vi "host_for_Tx_and_Rx_with scope.vi"() -> ()   [LabVIEW 2021]
uses:
  <vilib>/userdefined/High Color/nirio_resource_hc.ctl
  CTL/user config.ctl
  classes/5785_2_x_1600MHz/5785_2_x_1600MHz.lvclass
  <vilib>/Analysis/NI_AALBase.lvlib
  use with scope/states_for scope.ctl
  classes/device_type/device_type.lvclass
  <instrlib>/niScope/Acquire/Fetch/niScope Multi Fetch WDT.vi
  <instrlib>/niScope/Configure/Trigger/niScope Configure Trigger Edge.vi
  <vilib>/Analysis/1siggen.llb/Ramp Pattern by Delta.vi
  <instrlib>/niScope/Controls/niScope vertical coupling.ctl
  C:/Users/PXIe8108_Demo/Documents/CHAIM DATA/chaim/5785_sync_for_elbit/tx_pulse/pulse Tx Folder_lv_21/EMEA_ADG_EW_Multi_Emitter_Scenarios/classes/device_type/device_type.lvclass
  C:/Users/PXIe8108_Demo/Documents/CHAIM DATA/chaim/5785_sync_for_elbit/tx_pulse/pulse Tx Folder_lv_21/EMEA_ADG_EW_Multi_Emitter_Scenarios/classes/5785_2_x_1600MHz/5785_2_x_1600MHz.lvclass
panel:
  in  "scope cal file":path=path "C:/Users/PXIe8108_Demo/Documents/CHAIM DATA/chaim/5785_sync_for_elbit/tx_pulse/pulse Tx Folder_lv_21/EMEA_ADG_EW_Multi_Emitter_Scenarios/data/scope_cal_file.tdms"
  out "run number":i32
  in  "number of runs for test":dbl=5.0 format="%#_13g"
  in  "number of runs for cal":dbl=10.0 format="%#_13g"
  in  "read file":bool
  in  "save file":bool
  in  "file path":path=path "C:/Users/PXIe8108_Demo/Documents/CHAIM DATA/chaim/5785_sync_for_elbit/tx_pulse/pulse Tx Folder_lv_21/EMEA_ADG_EW_Multi_Emitter_Scenarios/data/cal_file.tdms"
  out "state":T1
  in  "cal":bool
  out "phase cal test (deg)":cluster{dbl[], dbl[]}[](graph)
  out "amp cal test(dB) 2":cluster{dbl[], dbl[]}[](graph)
  in  "cal mode":bool=TRUE
  in  "connection table (cannels 1,2,3 only)":dbl[](array[numeric])=[5.0, 2.0, 3.0]
  out "delta phase(deg)":cluster{dbl[], dbl[]}[](graph)
  out "delta amp (dB)":cluster{dbl[], dbl[]}[](graph)
  out "working":bool
  in  "Channel Name":string="0,1,2,3"
  in  "Resource Name":refnum<k15>="scope1" caption="Resource Name(s)"
  in  "pulse amplitude (dB)":dbl=-40.0 format="%#_13g"
  in  "pulse duration (s)":dbl=0.0002 format="%#_13p"
  in  "frequncy comb":cluster{"start":dbl, "end":dbl, "delta":dbl}={"start"=5000000.0, "end"=300000000.0, "delta"=500000.0} {"delta" format="%#_6p"; "end" format="%#_6p"; "start" format="%#_6p"}
  in  "devicess":T2[](array[typedef])=["5785_00", "5785_01", "5785_02"]
  # "5785 system alignment"
  # "RF setup"
  # "Cal Data"
  # "HW setup"
  # "scope mapping:\nchannel 0 => 5785_02 _0 \nchannel 1 => 5785_01 _0 \nchannel 2 => 5785_01 _1 \nchannel 3 => 5785_00 _1"
  # "Cal test"
  # "SW setup"
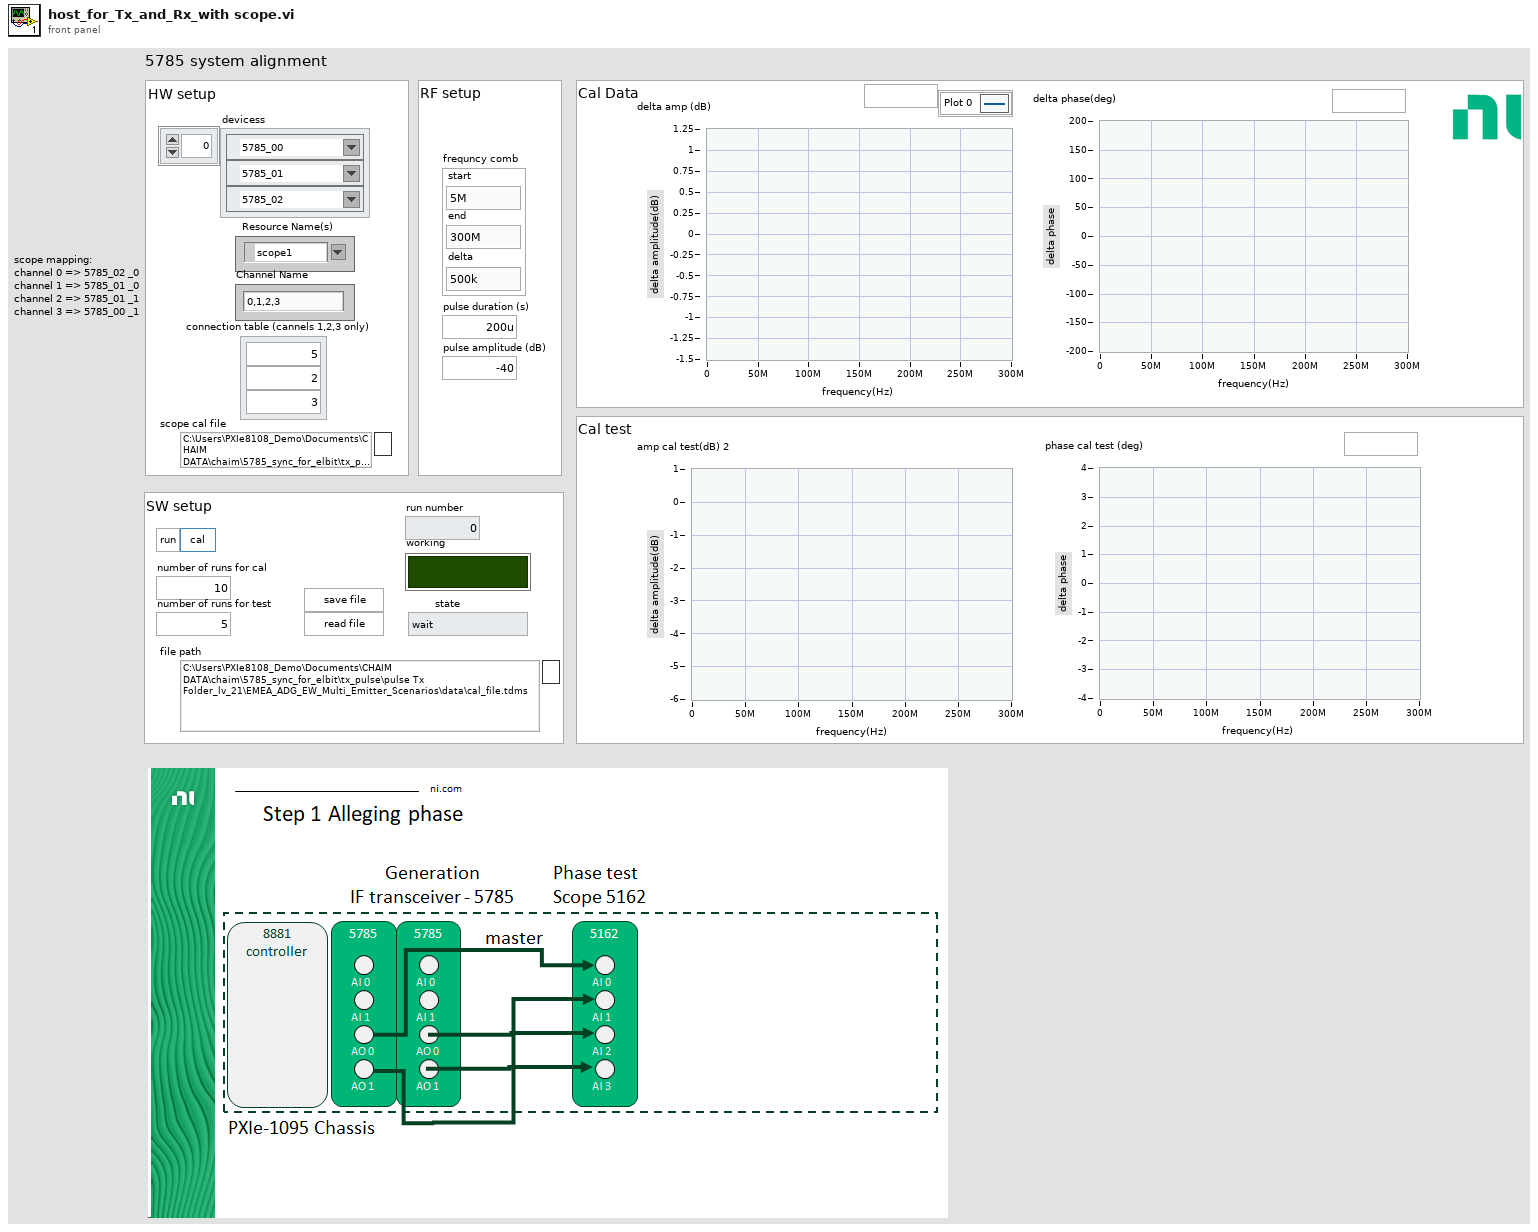
[diagram p1: front panel]
types:
  T1 = typedef "states_for scope.ctl" = enum16{"wait", "update ME config", "gen secenario", "INI ME", "INI scope", "trig", "close ME", "run mesearment", "save cal data", "get file data", "gen PDW file", "keep the data", "reset memory data", "prime the fifo"}
  T2 = typedef "nirio_resource_hc.ctl" = tag
  T3 = cluster{"freqency":dbl[], "phase":dbl[], "amp":dbl[]}
  T4 = enum16{"open", "open or create", "create or replace", "create", "open (read-only)"}
  T5 = typedef "user config.ctl" = cluster{"vst_device":refnum<k15>[], "RF gain ":dbl, "buffer size":u32, "center frequency (Hz) ":dbl, "P2P sample rate":dbl, "mode":enum16{"USRP - 180MHz", "5785 - 2*180MHz", "5785 - 3.2GHz", "P2P - VST"}, "devicess":T2[], "gen for df":bool, "Rx settings":cluster{"min PW         ":dbl, "max gap        ":dbl, "detection bar":dbl, "peak detect                        ":bool}, "use arb files":bool}
  T6 = typedef "states_for scope.ctl" = enum16{"wait", "update ME config", "gen secenario", "INI ME", "INI scope", "sync and trig", "close ME", "run mesearment", "save cal data", "get file data", "gen PDW file", "keep the data", "reset memory data"}
  T7 = cluster{"freqency":dbl[], "phase":dbl[], "amp":dbl[]}[]
  T8 = typedef "niScope vertical coupling.ctl" = i32
  T9 = typedef "PDW_lv2.ctl" = cluster{"t start":dbl, "frequency (Hz)":dbl, "duration (sec)":dbl, "mod type":T10, "mod depth":dbl, "phase (rad)":dbl[], "amp (lin)":dbl[], "trig":bool}
  T10 = typedef "mode_type.ctl" = enum8{"CW", "from memory 1", "NC - cw", "LFM", "BPSK", "QPSK"}
  T11 = typedef "PDW_lv2.ctl" = cluster{"t start":dbl, "frequency (Hz)":dbl, "duration (sec)":dbl, "mod type":T10, "mod depth":dbl, "trig":bool, "amp (lin)":dbl, "diraction (deg)":dbl, "phase(deg)":dbl}
  T12 = cluster{"frequncy":dbl, "d amp":dbl, "d phase":dbl}[]
  T13 = cluster{"frequncy":dbl, "d amp":dbl, "d phase":dbl}[][]
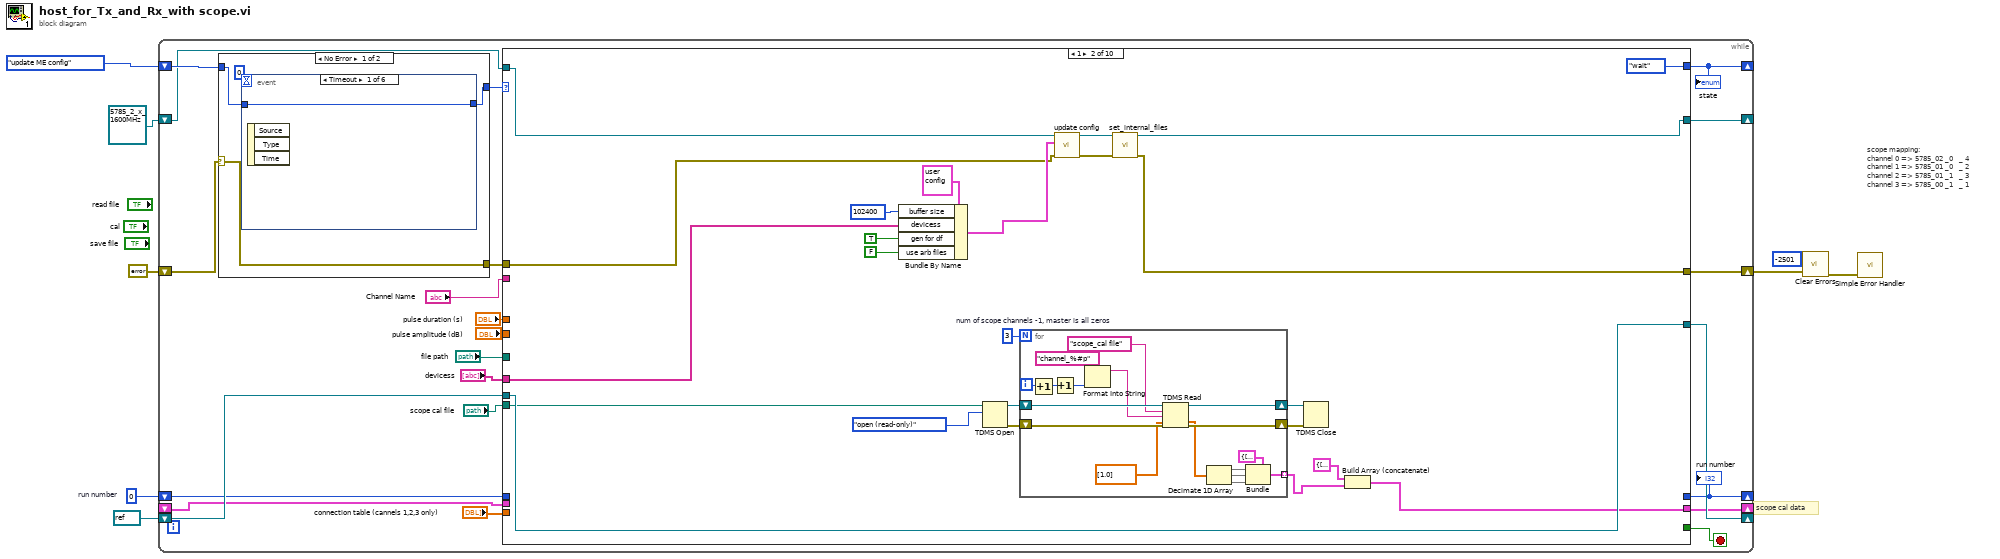
[diagram p0: block diagram]
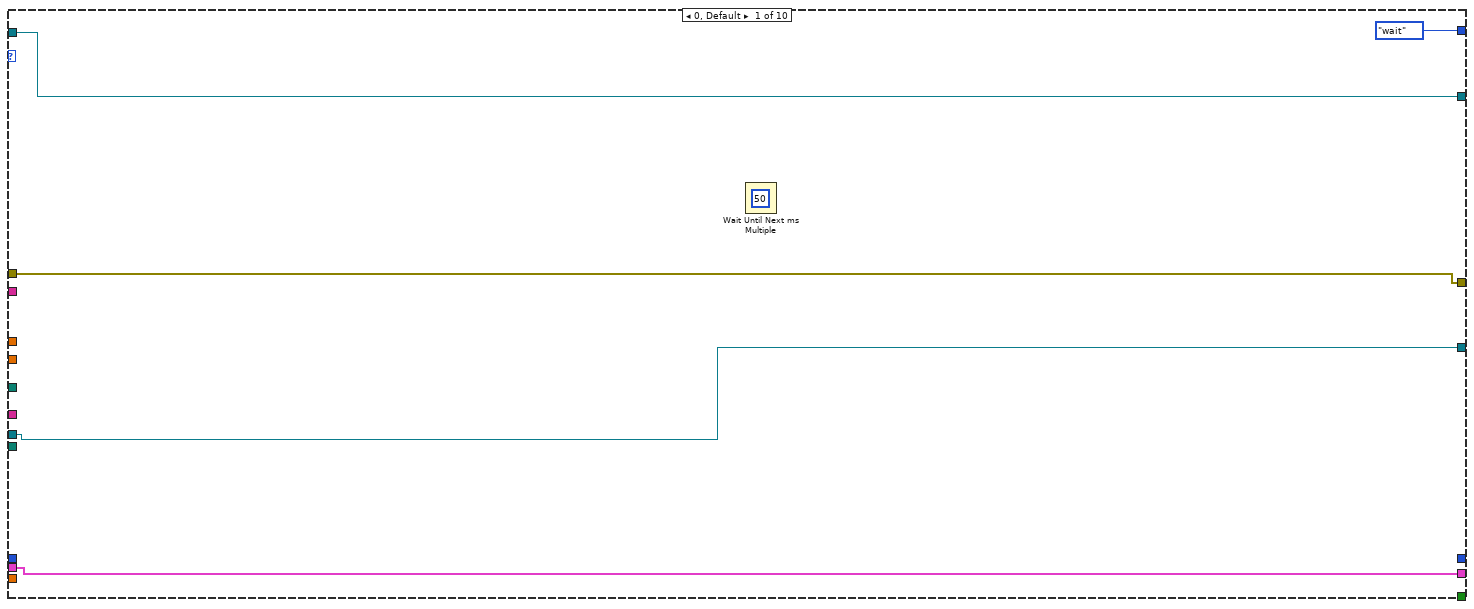
[diagram p2: hidden frame]
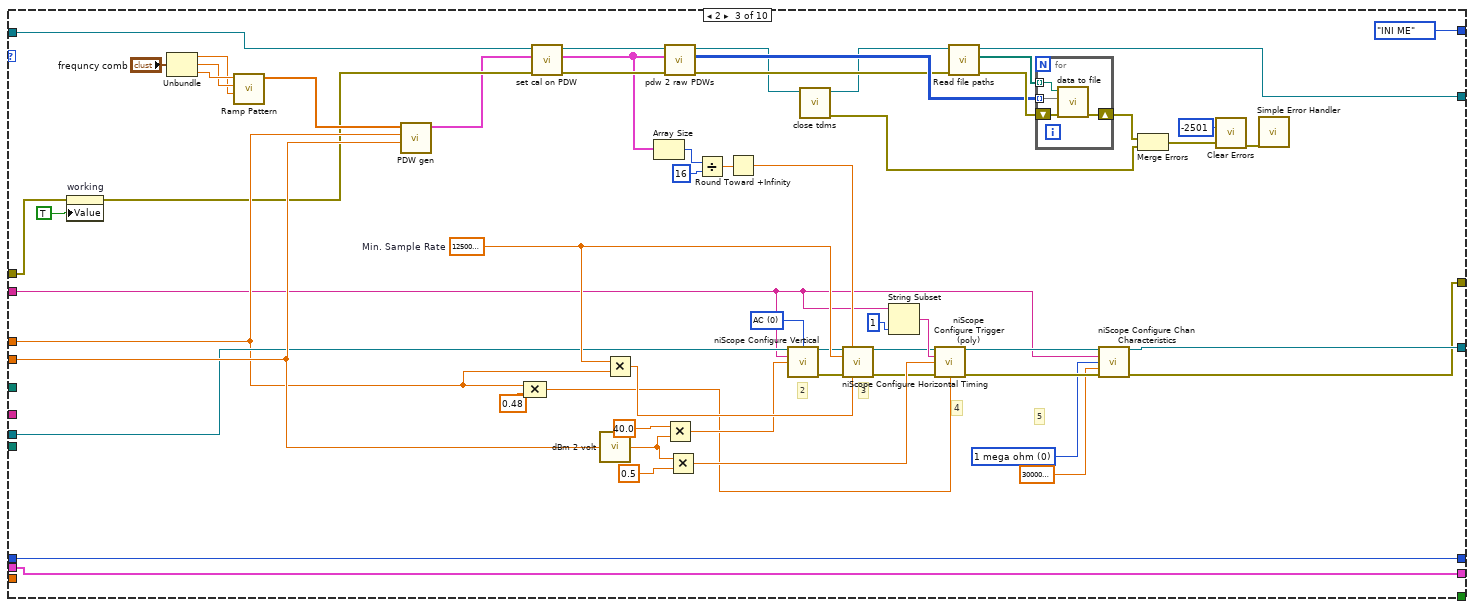
[diagram p3: hidden frame]
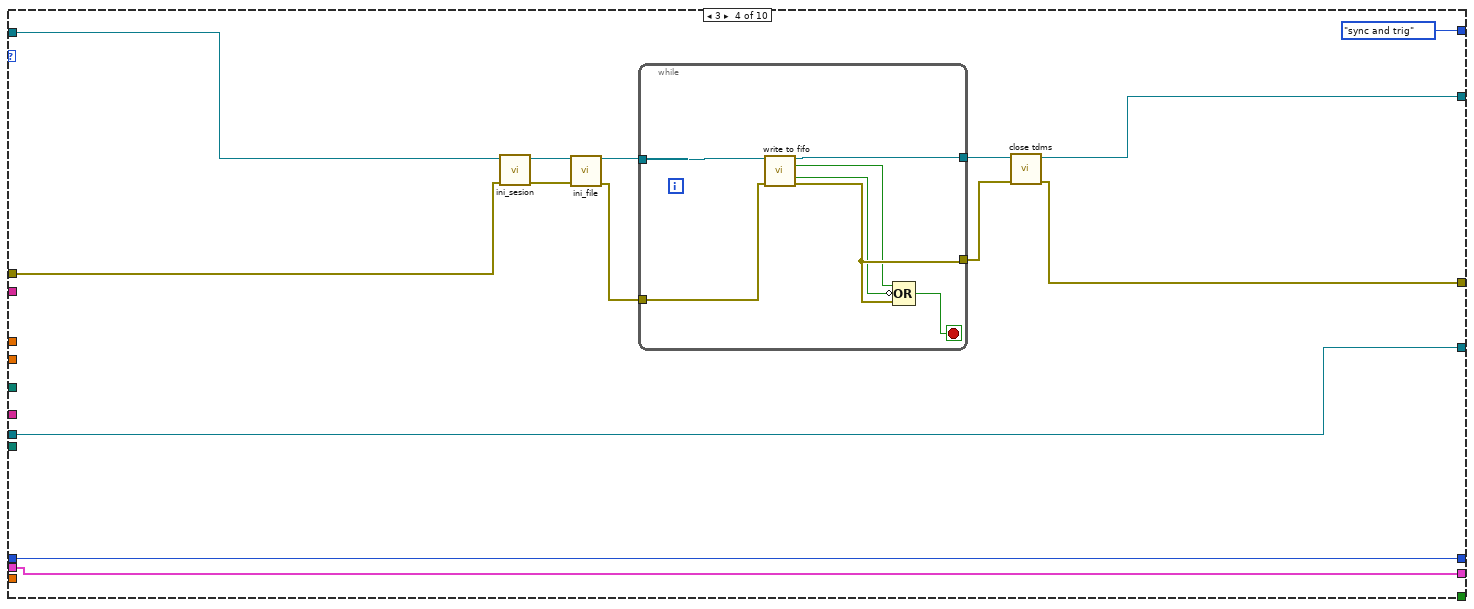
[diagram p4: hidden frame]
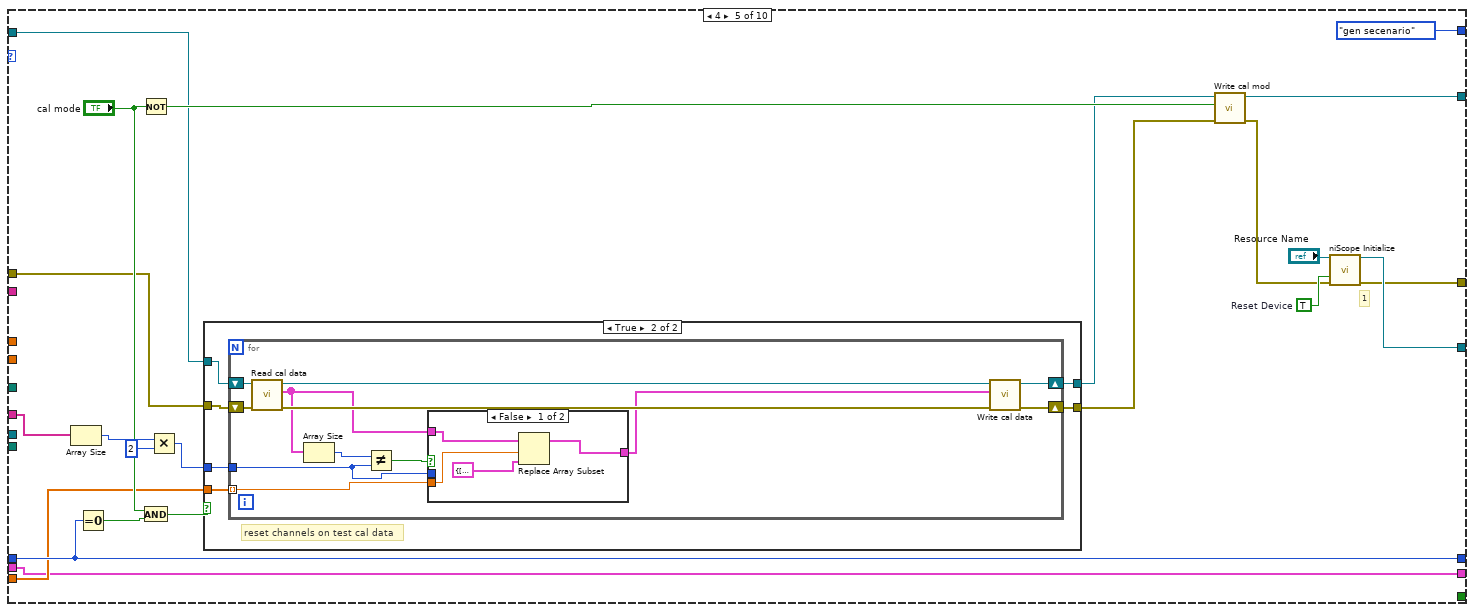
[diagram p5: hidden frame]
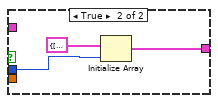
[diagram p7: hidden frame]
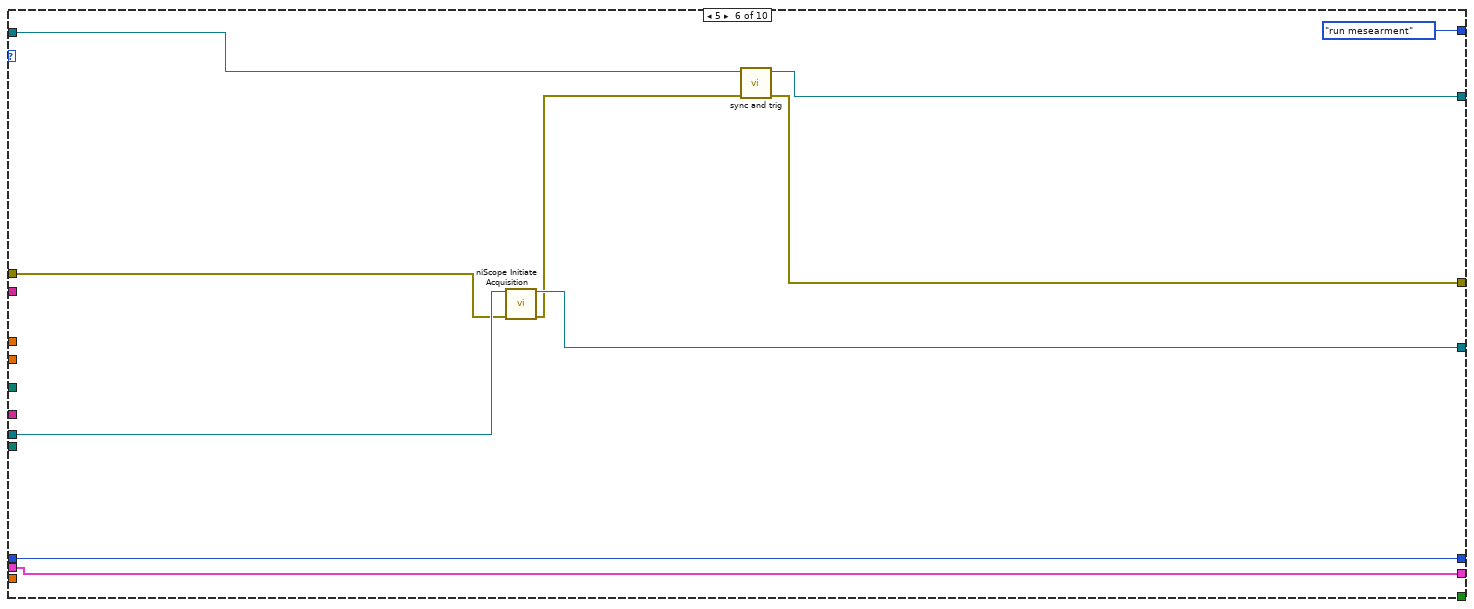
[diagram p8: hidden frame]
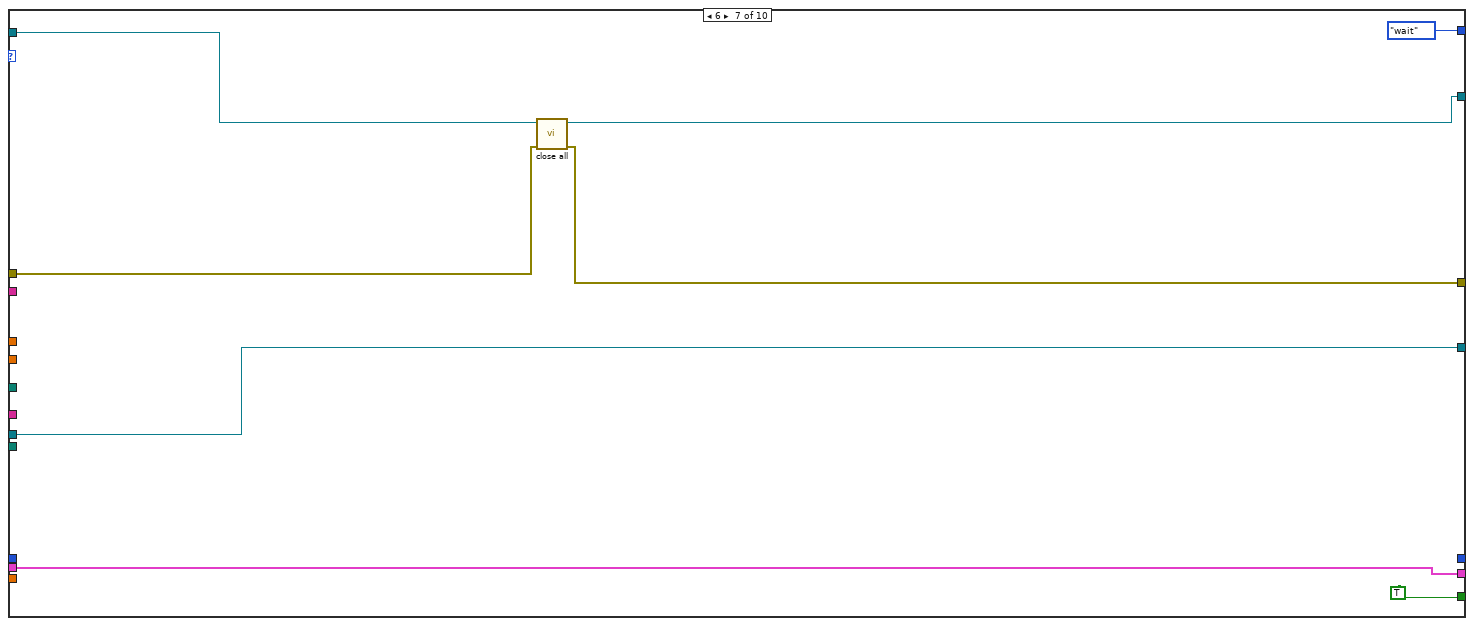
[diagram p9: hidden frame]
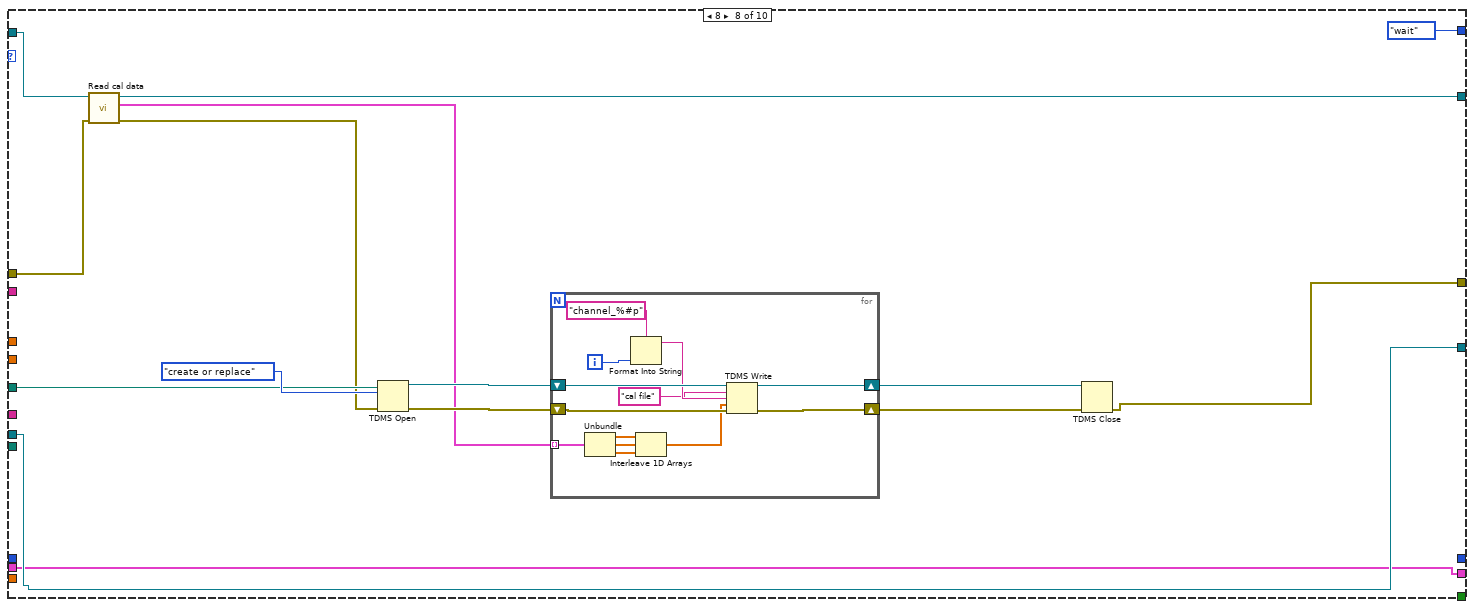
[diagram p10: hidden frame]
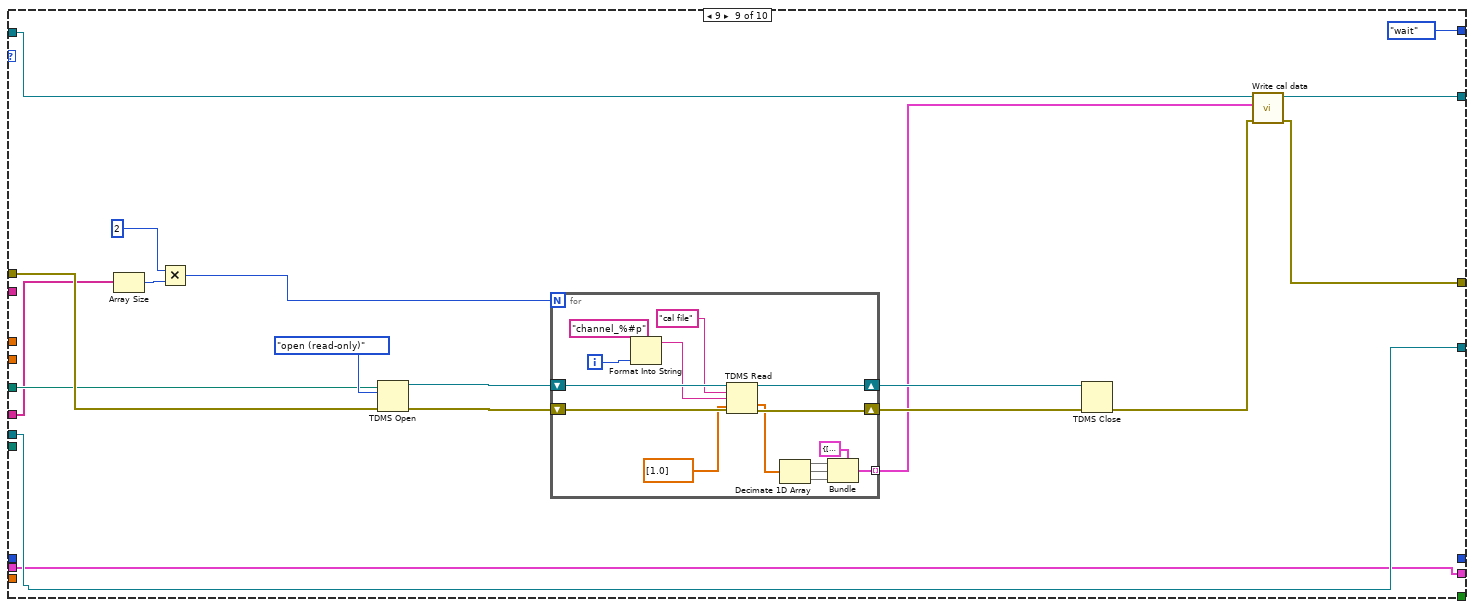
[diagram p11: hidden frame]
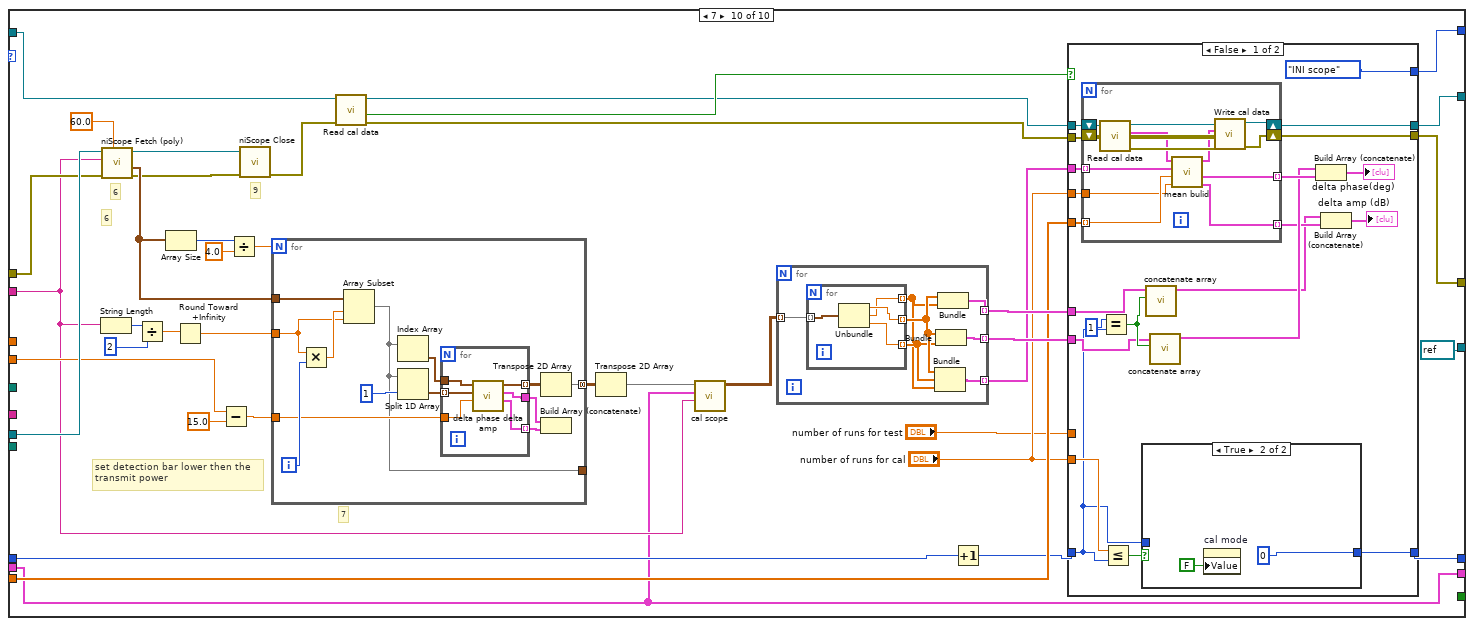
[diagram p12: hidden frame]
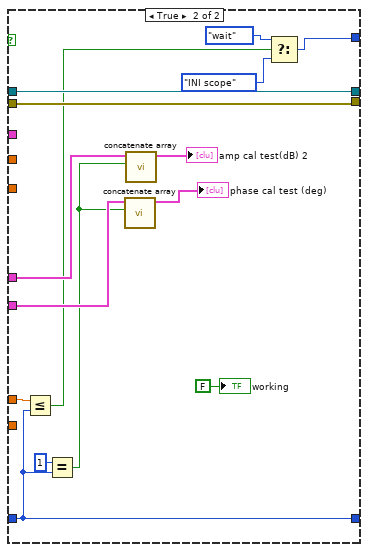
[diagram p14: hidden frame]
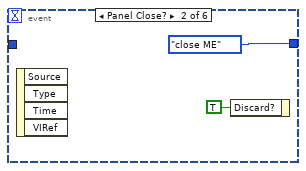
[diagram p15: hidden frame]
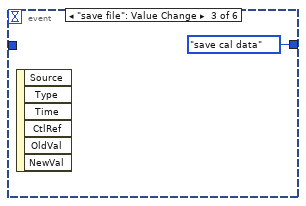
[diagram p16: hidden frame]
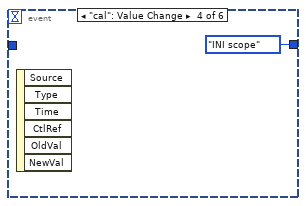
[diagram p17: hidden frame]
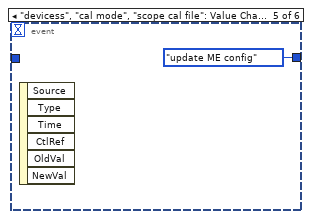
[diagram p18: hidden frame]
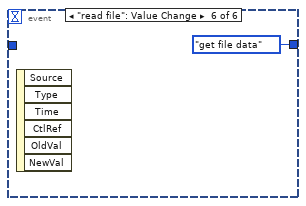
[diagram p19: hidden frame]
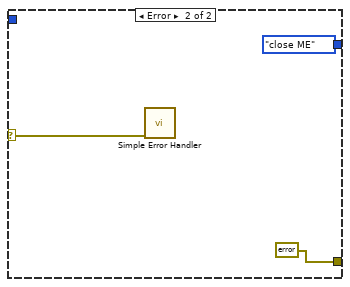
[diagram p20: hidden frame]
diagram:
  (unwired) -2501 ("specific error code to clear (0: all)")
  w3 = 0  # run number
  # "scope cal data"
  # "scope mapping:\nchannel 0 => 5785_02 _0   _ 4\nchannel 1 => 5785_01 _0   _ 2 \nchannel 2 => 5785_01 _1   _ 3\nchannel 3 => 5785_00 _1   _ 1"
  n1 = while {
    shift-right: [w16] -> _
    shift-left: states_for_scope."update ME config" -> [w27]
    shift-right: [w24] -> w2
    shift-left: errorcluster {"status"=FALSE, "code"=0, "source"=""} ("error out") -> [w29]
    shift-right: [w21] -> _
    shift-left: refnum<k15> refnum ("instrument handle out") -> [w20]
    shift-right: [w25] -> _
    shift-left: refnum<class "5785_2_x_1600MHz.lvclass"> refnum ("5785_2_x_1600MHz.lvclass") -> [w18]
    shift-right: [w12] -> _
    shift-left: w3 -> [w13]
    shift-right: [w9] -> _
    shift-left: _ -> [w8]
    stop <- w17 stop-if-true
    n2 = case shown="No Error" w29 {
      selector: w29 -> [w414 w424]
      tunnel: [w412 states_for_scope."close ME"] -> w28
      tunnel: w27 -> [w413 _]
      tunnel: [w414 errorcluster {"status"=FALSE, "code"=0, "source"=""} ("error IO")] -> w26
      frame No Error {
        n3 = event shown="[0] Timeout" {
          selector: _ -> [_ _ _ _ _ _]
          dyn-events: _ -> [_ _ _ _ _ _]
          timeout: 0 -> [_ _ _ _ _ _]
          tunnel: w413 -> [w415 _ _ _ _ _]
          tunnel: [w415 states_for_scope."close ME" states_for_scope."save cal data" states_for_scope."INI scope" states_for_scope."update ME config" states_for_scope."get file data"] -> w412
          event Timeout {
            n4 = event-data() -> ()  [unwired: 1 in, 3 out]
          }
          event Panel Close? {
            n5 = event-data() -> ()  [unwired: 1 in, 4 out]
            n6 = event-data("Discard?"=TRUE) -> ()  [unwired: 1 in, 1 out]
          }
          event "save file": Value Change {
            n7 = event-data() -> ()  [unwired: 1 in, 6 out]
          }
          event "cal": Value Change {
            n8 = event-data() -> ()  [unwired: 1 in, 6 out]
          }
          event "devicess", "cal mode", "scope cal file": Value Change {
            n9 = event-data() -> ()  [unwired: 1 in, 6 out]
          }
          event "read file": Value Change {
            n10 = event-data() -> ()  [unwired: 1 in, 6 out]
          }
        }
      }
      frame Error {
        n11 = call <vilib>:"Simple Error Handler.vi"("error in (no error)"=w424) -> ()  [unwired: 4 in, 5 out]
      }
    }
    n12 = case shown="1" w28 {
      tunnel: w26 -> [w33 w50 w98 w147 w167 w214 w224 w229 w270 w316]
      tunnel: [w34 w48 w105 w140 w175 w212 w225 w231 w259 w308] -> w25
      tunnel: [w33 w47 w86 w141 w178 w215 w223 w235 w256 w310] -> w24
      tunnel: "pulse duration (s)" -> [_ _ w106 _ _ _ _ _ _ _]
      tunnel: "pulse amplitude (dB)" -> [_ _ w108 _ _ _ _ _ _ w311]
      tunnel: [w32 w52 w87 w146 w179 w217 w222 w240 w272 refnum<k15> refnum ("instrument handle out")] -> w21
      tunnel: w20 -> [w32 w52 w107 w146 _ w218 w222 w240 w272 w317]
      tunnel: "Channel Name" -> [_ _ w83 _ _ _ _ _ _ w290]
      tunnel: w18 -> [w34 w46 w95 w148 w172 w213 w226 w232 w260 w309]
      tunnel: [_ _ _ _ _ _ TRUE _ _ _] -> w17
      tunnel: [states_for_scope."wait" states_for_scope."wait" states_for_scope."INI ME" states_for_scope."sync and trig" states_for_scope."gen secenario" states_for_scope."run mesearment" states_for_scope."wait" states_for_scope."wait" states_for_scope."wait" w303] -> w16
      tunnel: "file path" -> [_ _ _ _ _ _ _ w233 w265 _]
      tunnel: "devicess" -> [_ w49 _ _ w163 _ _ _ w262 _]
      tunnel: w13 -> [_ _ w91 w144 w173 w210 _ _ _ w298]
      tunnel: [_ _ w91 w144 w173 w210 _ _ _ w300] -> w12
      tunnel: "connection table (cannels 1,2,3 only)" -> [_ _ _ _ w165 _ _ _ _ w302]
      tunnel: "scope cal file" -> [_ w39 _ _ _ _ _ _ _ _]
      tunnel: [w30 w36 w77 w139 w164 w209 w219 w227 w255 w289] -> w9
      tunnel: w8 -> [w30 _ w77 w139 w164 w209 w219 w227 w255 w289]
      frame 0, Default {
        n13 = Wait Until Next ms Multiple(millisecond multiple=u32 50) -> ()  [unwired: 1 out]
      }
      frame 1 {
        w41 = 3  # num of scope channels -1, master is all zeros
        n14 = Bundle By Name(cluster=T5 {"vst_device"=["VST_1", "VST_2"], "RF gain "=10.0, "buffer size"=524288, "center frequency (Hz) "=1000000000.0, "P2P sample rate"=200000000.0, "mode"=enum."5785 - 2*180MHz", "devicess"=["IF_transiver_0", "IF_transiver_1", "IF_transiver_2"], "gen for df"=FALSE, "Rx settings"={"min PW         "=0.0, "max gap        "=0.0, "detection bar"=0.0, "peak detect                        "=FALSE}, "use arb files"=TRUE} ("user configurations"), "buffer size"=u32 102400, "devicess"=w49, "gen for df"=TRUE, "use arb files"=FALSE) -> (w59:T5)
        n15 = TDMS Open(10:T4."open (read-only)" ("operation (0:open)"), 11:w39) -> (0:w43:errorcluster, 3:w42:refnum<k34>)  [unwired: 5 in]
        n16 = for {
          N: w41 -> [_]
          shift-right: [w74] -> w44
          shift-left: w42 -> [w76]
          shift-right: [w73] -> w45
          shift-left: w43 -> [w75]
          tunnel: [w63] -> w38 mode=indexing
          i -> [w62]
          n17 = Increment(x=w62) -> (x+1=w60:i32)
          n18 = Increment(x=w60) -> (x+1=w61:i32)
          n19 = Format Into String(format string="channel_%#p", w61) -> (resulting string=w71:string)  [unwired: 2 in, 1 out]
          n20 = TDMS Read(0:w76, 5:"scope_cal file" ("group name in (Untitled)"), 7:w71, 11:w75, 12:dbl[] [1.0] ("interleaved array")) -> (4:w74:refnum<k34>, 10:w68:dbl[], 15:w73:errorcluster)  [unwired: 3 in, 3 out]
          n21 = Decimate 1D Array(w68) -> (w66:dbl[], w65:dbl[], w64:dbl[])
          n22 = Bundle(cluster=T3 {"freqency"=[], "phase"=[], "amp"=[]}, "freqency"=w66, "phase"=w65, "amp"=w64) -> (w63:T3)
        }
        n23 = call-dynamic "update config.vi"("error in (no error)"=w50, "user configurations"=w59, "5785_2_x_1600MHz in"=w46) -> ("error out"=w57:errorcluster, "5785_2_x_1600MHz out"=w58:refnum<class "5785_2_x_1600MHz.lvclass">)  [unwired: 5 in, 2 out]
        n24 = call-dynamic "set_internal_files.vi"("error in (no error)"=w57, "device_type in"=w58) -> ("error out"=w47:errorcluster, "device_type out"=w48:refnum<class "5785_2_x_1600MHz.lvclass">)  [unwired: 8 in]
        n25 = TDMS Close(8:w45, 11:w44) -> ()  [unwired: 2 out]
        n26 = Build Array (concatenate)(T3 {"freqency"=[], "phase"=[], "amp"=[]}, w38) -> (w36:T7)
      }
      frame 2 {
        w85 = u32 0 items=["1 mega ohm"=0, "50 ohms"=2] ("input impedance")
        w90 = T8 0 items=["AC", "DC", "Ground"] ("vertical coupling")
        w114 = 1250000000.0  # Min. Sample Rate
        # "5"
        # "4"
        # "3"
        # "2"
        n27 = property on="working" class="Bool (strict)"(error in=w98, "Value"=TRUE ("done")) -> (error out=w94:errorcluster)  [unwired: 1 in, 1 out]
        n28 = Unbundle("frequncy comb") -> ("start"=w129:dbl, "end"=w130:dbl, "delta"=w131:dbl)
        n29 = call-poly <vilib>:"Ramp Pattern.vi"("start"=w129, "end"=w130, "delta"=w131) -> ("Ramp Pattern"=w132:dbl[])  [unwired: 6 in, 2 out]
        n30 = call "PDW gen.vi"("pulse amplitude"=w108, "pulse duration"=w106, "frequency list"=w132) -> ("PDW out"=w93:T9[])  [unwired: 7 in, 1 out]
        n31 = Compound Arithmetic op=MULTIPLY(w106, 0.48 ("value")) -> (w118:dbl)
        n32 = call "set cal on PDW.vi"("error in (no error)"=w94, "PDWs on channels"=w93, "device_type in"=w95) -> ("error out"=w96:errorcluster, "PDWs on channels"=w92:cluster{T11[]}[], "device_type out"=w97:refnum<class "5785_2_x_1600MHz.lvclass">)  [unwired: 6 in]
        n33 = call "dBm 2 volt.vi"("dBm"=w108) -> ("V"=w119:dbl)
        n34 = Multiply(x=w114, y=w106) -> (x*y=w122:dbl)
        n35 = Array Size(array=w92) -> (size(s)=w133:i32)
        n36 = call-dynamic "pdw 2 raw PDWs.vi"("error in (no error)"=w96, "PDWs on channels"=w92, "device_type in"=w97) -> ("error out"=w124:errorcluster, "Array"=w126:u64[][], "device_type out"=w101:refnum<class "5785_2_x_1600MHz.lvclass">)  [unwired: 6 in]
        n37 = Multiply(x=40.0, y=w119) -> (x*y=w121:dbl)
        n38 = Multiply(x=w119, y=0.5) -> (x*y=w120:dbl)
        n39 = Divide(x=w133, y=16) -> (x/y=w134:dbl)
        n40 = Round Toward +Infinity(x=w134) -> (ceil(x): smallest int >= x=w109:dbl)
        n41 = call <instrlib>:"niScope Configure Vertical.vi"("instrument handle"=w107, "vertical coupling"=w90, "channels"=w83, "vertical range"=w121) -> ("instrument handle out"=w103:refnum<k15>, "error out"=w102:errorcluster)  [unwired: 10 in]
        n42 = call-dynamic "close tdms.vi"("device_type in"=w101) -> ("error out"=w80:errorcluster, "device_type out"=w100:refnum<class "5785_2_x_1600MHz.lvclass">)  [unwired: 9 in]
        n43 = call <instrlib>:"niScope Configure Horizontal Timing.vi"("instrument handle"=w103, "number of records"=w109, "min sample rate"=w114, "error in"=w102, "min record length"=w122) -> ("instrument handle out"=w116:refnum<k15>, "error out"=w115:errorcluster)  [unwired: 9 in]
        n44 = String Subset(string=w83, length (rest)=1 ("length (rest)")) -> (substring=w117:string)  [unwired: 1 in]
        n45 = call-poly <instrlib>:"niScope Configure Trigger (poly).vi"("instrument handle"=w116, "trigger source"=w117, "trigger level"=w120, "error in"=w115, "trigger delay"=w118) -> ("instrument handle out"=w89:refnum<k15>, "error out"=w88:errorcluster)  [unwired: 9 in]
        n46 = call-dynamic "Read file paths.vi"("error in (no error)"=w124, "device_type in"=w100) -> ("error out"=w127:errorcluster, "file paths"=w125:path[], "device_type out"=w105:refnum<class "5785_2_x_1600MHz.lvclass">)  [unwired: 6 in, 1 out]
        n47 = for {
          tunnel: w126 -> [w136] mode=indexing
          shift-right: [w137] -> w81
          shift-left: w127 -> [w138]
          tunnel: w125 -> [w135] mode=indexing
          n48 = call "data to file.vi"("error in (no error)"=w138, "Array"=w136, "Path"=w135) -> ("error out"=w137:errorcluster)  [unwired: 8 in]
        }
        n49 = call <instrlib>:"niScope Configure Chan Characteristics.vi"("instrument handle"=w89, "channels"=w83, "input impedance"=w85, "maximum input frequency"=300000000.0, "error in"=w88) -> ("instrument handle out"=w87:refnum<k15>, "error out"=w86:errorcluster)  [unwired: 9 in]
        n50 = Merge Errors(w81, w80) -> (w79:errorcluster)
        n51 = call <vilib>:"Clear Errors.vi"("error in (no error)"=w79, "specific error code to clear (0: all)"=-2501) -> ("error out"=w78:errorcluster)  [unwired: 4 in, 1 out]
        n52 = call <vilib>:"Simple Error Handler.vi"("error in (no error)"=w78) -> ()  [unwired: 4 in, 5 out]
      }
      frame 3 {
        n53 = call-dynamic "ini_sesion.vi"("error in (no error)"=w147, "5785_2_x_1600MHz in"=w148) -> ("error out"=w150:errorcluster, "5785_2_x_1600MHz out"=w149:refnum<class "5785_2_x_1600MHz.lvclass">)  [unwired: 8 in]
        n54 = call-dynamic "ini_file.vi"("device_type in"=w149, "error in (no error)"=w150) -> ("device_type out"=w151:refnum<class "5785_2_x_1600MHz.lvclass">, "error out"=w152:errorcluster)  [unwired: 11 in, 1 out]
        n55 = while {
          tunnel: w151 -> [w159]
          tunnel: w152 -> [w158]
          tunnel: [w157] -> w143
          tunnel: [w155] -> w142
          stop <- w156 stop-if-true
          n56 = call-dynamic "write to fifo.vi"("5785_2_x_1600MHz in"=w159, "error in (no error)"=w158) -> ("5785_2_x_1600MHz out"=w157:refnum<class "5785_2_x_1600MHz.lvclass">, "done write file"=w153:bool, "room on fifo"=w154:bool, "error out"=w155:errorcluster)  [unwired: 9 in, 1 out]
          n57 = Compound Arithmetic op=OR(w153, invert w154, w155) -> (w156:bool)
        }
        n58 = call-dynamic "close tdms.vi"("error in (no error)"=w142, "device_type in"=w143) -> ("error out"=w141:errorcluster, "device_type out"=w140:refnum<class "5785_2_x_1600MHz.lvclass">)  [unwired: 8 in]
      }
      frame 4 {
        w180 = TRUE  # Reset Device
        # "1"
        n59 = Array Size(array=w163) -> (size(s)=w162:i32)
        n60 = Equal To 0?(x=w173) -> (x = 0?=w169:bool)
        n61 = Not(x="cal mode") -> (.not. x?=w176:bool)
        n62 = And(x="cal mode", y=w169) -> (x .and. y?=w168:bool)
        n63 = Multiply(x=w162, y=2) -> (x*y=w160:i32)
        n64 = case shown="True" w168 {
          tunnel: w172 -> [w183 w189]
          tunnel: [w183 w188] -> w171
          tunnel: w167 -> [w182 w187]
          tunnel: [w182 w186] -> w166
          tunnel: w165 -> [_ w185]
          tunnel: w160 -> [_ w184]
          frame False {
          }
          frame True {
            # "reset channels on test cal data"
            n65 = for {
              shift-right: [w198] -> w188
              shift-left: w189 -> [w199]
              shift-right: [w196] -> w186
              shift-left: w187 -> [w197]
              tunnel: w185 -> [w191] mode=indexing
              tunnel: w184 -> [w190]
              n66 = call-dynamic "Read cal data.vi"("error in (no error)"=w197, "device_type in"=w199) -> ("error out"=w200:errorcluster, "cal data"=w194:T7, "device_type out"=w201:refnum<class "5785_2_x_1600MHz.lvclass">)  [unwired: 6 in, 1 out]
              n67 = Array Size(array=w194) -> (size(s)=w193:i32)
              n68 = Not Equal?(x=w193, y=w190) -> (x != y?=w192:bool)
              n69 = case shown="False" w192 {
                tunnel: w194 -> [w205 _]
                tunnel: [w204 w208] -> w195
                tunnel: w191 -> [w203 _]
                tunnel: w190 -> [_ w206]
                frame False {
                  n70 = Replace Array Subset(array=w205, new element=T3 {"freqency"=[], "phase"=[], "amp"=[]} ("new element/subarray"), index=w203) -> (w204:T7)
                }
                frame True {
                  n71 = Initialize Array(cluster{dbl[], dbl[], dbl[]} {[], [], []} ("new element/subarray"), w206) -> (w208:cluster{dbl[], dbl[], dbl[]}[])
                }
              }
              n72 = call-dynamic "Write cal data.vi"("error in (no error)"=w200, "cal data"=w195, "device_type in"=w201) -> ("error out"=w196:errorcluster, "device_type out"=w198:refnum<class "5785_2_x_1600MHz.lvclass">)  [unwired: 7 in]
            }
          }
        }
        n73 = call-dynamic "Write cal mod.vi"("error in (no error)"=w166, "apply cal data"=w176, "device_type in"=w171) -> ("error out"=w174:errorcluster, "device_type out"=w175:refnum<class "5785_2_x_1600MHz.lvclass">)  [unwired: 7 in]
        n74 = call <instrlib>:"niScope Initialize.vi"("resource name"="Resource Name", "reset device"=w180, "error in"=w174) -> ("instrument handle"=w179:refnum<k15>, "error out"=w178:errorcluster)  [unwired: 11 in]
      }
      frame 5 {
        n75 = call <instrlib>:"niScope Initiate Acquisition.vi"("instrument handle"=w218, "error in"=w214) -> ("instrument handle out"=w217:refnum<k15>, "error out"=w216:errorcluster)  [unwired: 12 in]
        n76 = call-dynamic "sync and trig.vi"("error in (no error)"=w216, "device_type in"=w213) -> ("error out"=w215:errorcluster, "device_type out"=w212:refnum<class "5785_2_x_1600MHz.lvclass">)  [unwired: 8 in]
      }
      frame 6 {
        n77 = call-dynamic "close all.vi"("error in (no error)"=w224, "5785_2_x_1600MHz in"=w226) -> ("error out"=w223:errorcluster, "5785_2_x_1600MHz out"=w225:refnum<class "5785_2_x_1600MHz.lvclass">)  [unwired: 8 in]
      }
      frame 8 {
        n78 = call-dynamic "Read cal data.vi"("error in (no error)"=w229, "device_type in"=w232) -> ("error out"=w228:errorcluster, "cal data"=w230:T7, "device_type out"=w231:refnum<class "5785_2_x_1600MHz.lvclass">)  [unwired: 6 in, 1 out]
        n79 = TDMS Open(8:w228, 10:T4."create or replace" ("operation (0:open)"), 11:w233) -> (0:w238:errorcluster, 3:w239:refnum<k34>)  [unwired: 4 in]
        n80 = for {
          shift-right: [w252] -> w237
          shift-left: w239 -> [w254]
          shift-right: [w251] -> w236
          shift-left: w238 -> [w253]
          tunnel: w230 -> [w245] mode=indexing
          i -> [w249]
          n81 = Unbundle(w245) -> ("freqency"=w244:dbl[], "phase"=w243:dbl[], "amp"=w242:dbl[])
          n82 = Format Into String(format string="channel_%#p", w249) -> (resulting string=w247:string)  [unwired: 2 in, 1 out]
          n83 = Interleave 1D Arrays(w244, w243, w242) -> (w250:dbl[])
          n84 = TDMS Write(0:w254, 5:"cal file" ("group name in (Untitled)"), 7:w247, 9:w250, 11:w253) -> (4:w252:refnum<k34>, 15:w251:errorcluster)  [unwired: 1 in, 2 out]
        }
        n85 = TDMS Close(8:w236, 11:w237) -> (0:w235:errorcluster)  [unwired: 1 out]
      }
      frame 9 {
        n86 = Array Size(array=w262) -> (size(s)=w264:i32)
        n87 = Multiply(x=2, y=w264) -> (x*y=w261:i32)
        n88 = TDMS Open(8:w270, 10:T4."open (read-only)" ("operation (0:open)"), 11:w265) -> (0:w269:errorcluster, 3:w271:refnum<k34>)  [unwired: 4 in]
        n89 = for {
          N: w261 -> [_]
          shift-right: [w286] -> w268
          shift-left: w271 -> [w288]
          shift-right: [w285] -> w267
          shift-left: w269 -> [w287]
          tunnel: [w274] -> w258 mode=indexing
          i -> [w284]
          n90 = Format Into String(format string="channel_%#p", w284) -> (resulting string=w282:string)  [unwired: 2 in, 1 out]
          n91 = TDMS Read(0:w288, 5:"cal file" ("group name in (Untitled)"), 7:w282, 11:w287, 12:dbl[] [1.0] ("interleaved array")) -> (4:w286:refnum<k34>, 10:w279:dbl[], 15:w285:errorcluster)  [unwired: 3 in, 3 out]
          n92 = Decimate 1D Array(w279) -> (w277:dbl[], w276:dbl[], w275:dbl[])
          n93 = Bundle(cluster=T3 {"freqency"=[], "phase"=[], "amp"=[]}, "freqency"=w277, "phase"=w276, "amp"=w275) -> (w274:T3)
        }
        n94 = TDMS Close(8:w267, 11:w268) -> (0:w257:errorcluster)  [unwired: 1 out]
        n95 = call-dynamic "Write cal data.vi"("error in (no error)"=w257, "cal data"=w258, "device_type in"=w260) -> ("error out"=w256:errorcluster, "device_type out"=w259:refnum<class "5785_2_x_1600MHz.lvclass">)  [unwired: 7 in]
      }
      frame 7 {
        # "set detection bar lower then the\ntransmit power"
        # "6"
        # "9"
        # "7"
        # "6"
        n96 = String Length(string=w290) -> (length=w296:i32)
        n97 = call-poly <instrlib>:"niScope Fetch (poly).vi"("timeout"=60.0, "error in"=w316, "channels"=w290, "instrument handle"=w317) -> ("error out"=w322:errorcluster, "wfm"=w326:waveform(dbl)[], "instrument handle out"=w321:refnum<k15>)  [unwired: 4 in, 1 out]
        n98 = Divide(x=w296, y=2) -> (x/y=w294:dbl)
        n99 = Array Size(array=w326) -> (size(s)=w323:i32)
        n100 = Round Toward +Infinity(x=w294) -> (ceil(x): smallest int >= x=w293:dbl)
        n101 = Subtract(x=w311, y=15.0) -> (x-y=w325:dbl)
        n102 = Divide(x=w323, y=4.0) -> (x/y=w324:dbl)
        n103 = call <instrlib>:"niScope Close.vi"("instrument handle"=w321, "error in"=w322) -> ("error out"=w307:errorcluster)  [unwired: 13 in]
        n104 = for {
          N: w324 -> [_]
          tunnel: w326 -> [w393]
          tunnel: w325 -> [w387]
          tunnel: [w385] -> w327 mode=concatenating
          tunnel: [w384] -> _
          tunnel: w293 -> [w381]
          i -> [w392]
          n105 = Multiply(x=w381, y=w392) -> (x*y=w391:dbl)
          n106 = Array Subset(array=w393, index=w391, length=w381) -> (w384:waveform(dbl)[])
          n107 = Index Array(array=w384) -> (element=w389:waveform(dbl))  [unwired: 1 in]
          n108 = Split 1D Array(array=w384, index=1) -> (second subarray=w388:waveform(dbl)[])  [unwired: 1 out]
          n109 = for {
            tunnel: w389 -> [w399]
            tunnel: w388 -> [w398] mode=indexing
            tunnel: w387 -> [w397]
            tunnel: [w396] -> w386 mode=indexing
            tunnel: [w395] -> w383
            tunnel: [w394] -> w382 mode=indexing
            n110 = call "delta phase delta amp.vi"("detection bar"=w397, "signal in 2"=w398, "signal in 1"=w399) -> ("PSD 1"=w394:cluster{"f0":dbl, "df":dbl, "magnitude":dbl[]}, "PSD 0"=w395:cluster{"f0":dbl, "df":dbl, "magnitude":dbl[]}, "cal data"=w396:T12)  [unwired: 6 in]
          }
          n111 = Transpose 2D Array(2D array=w386) -> (transposed array=w385:T13)
          n112 = Build Array (concatenate)(w383, w382) -> ()  [unwired: 1 out]
        }
        n113 = call-dynamic "Read cal data.vi"("error in (no error)"=w307, "device_type in"=w309) -> ("error out"=w304:errorcluster, "apply cal data"=w306:bool, "device_type out"=w305:refnum<class "5785_2_x_1600MHz.lvclass">)  [unwired: 6 in, 1 out]
        n114 = Transpose 2D Array(2D array=w327) -> (transposed array=w292:T13)
        n115 = call "cal scope.vi"("Channel Name"=w290, "scope cal data"=w289, "measured data"=w292) -> ("measured and cal data"=w291:T13)  [unwired: 8 in]
        n116 = for {
          tunnel: w291 -> [w406] mode=indexing
          tunnel: [w405] -> w314 mode=indexing
          tunnel: [w404] -> w313 mode=indexing
          tunnel: [w400] -> w312 mode=indexing
          n117 = for {
            tunnel: w406 -> [w410] mode=indexing
            tunnel: [w409] -> w403 mode=indexing
            tunnel: [w408] -> w402 mode=indexing
            tunnel: [w407] -> w401 mode=indexing
            n118 = Unbundle(w410) -> ("frequncy"=w409:dbl, "d amp"=w407:dbl, "d phase"=w408:dbl)
          }
          n119 = Bundle(w403, w402, w401) -> (w400:cluster{dbl[], dbl[], dbl[]})  [unwired: 1 in]
          n120 = Bundle(w403, w402) -> (w404:cluster{dbl[], dbl[]})  [unwired: 1 in]
          n121 = Bundle(w403, w401) -> (w405:cluster{dbl[], dbl[]})  [unwired: 1 in]
        }
        n122 = Increment(x=w298) -> (x+1=w297:i32)
        n123 = case shown="False" w306 {
          tunnel: w312 -> [w349 _]
          tunnel: w302 -> [w348 _]
          tunnel: w314 -> [w339 w377]
          tunnel: w313 -> [w337 w375]
          tunnel: w305 -> [w347 w379]
          tunnel: w304 -> [w346 w378]
          tunnel: [w345 w378] -> w310
          tunnel: [w344 w379] -> w308
          tunnel: [states_for_scope."INI scope" w371] -> w303
          tunnel: "number of runs for cal" -> [w342 _]
          tunnel: w297 -> [w329 w372]
          tunnel: "number of runs for cal" -> [w330 _]
          tunnel: [w340 w372] -> w300
          tunnel: "number of runs for test" -> [_ w367]
          frame False {
            n124 = for {
              tunnel: w349 -> [w357] mode=indexing
              tunnel: w348 -> [w358] mode=indexing
              shift-right: [w363] -> w344
              shift-left: w347 -> [w365]
              shift-right: [w360] -> w345
              shift-left: w346 -> [w362]
              tunnel: w342 -> [w356]
              tunnel: [w354] -> w335 mode=indexing
              tunnel: [w353] -> w333 mode=indexing
              n125 = call-dynamic "Read cal data.vi"("error in (no error)"=w362, "device_type in"=w365) -> ("error out"=w361:errorcluster, "cal data"=w359:T7, "device_type out"=w364:refnum<class "5785_2_x_1600MHz.lvclass">)  [unwired: 6 in, 1 out]
              n126 = call "mean bulid.vi"("mean factor"=w356, "channel"=w358, "new data"=w357, "memory data"=w359) -> ("amp cal"=w353:cluster{"freqency":dbl[], "Array":dbl[]}, "phase cal"=w354:cluster{"freqency":dbl[], "Array":dbl[]}, "memory data"=w355:T7)  [unwired: 5 in]
              n127 = call-dynamic "Write cal data.vi"("error in (no error)"=w361, "cal data"=w355, "device_type in"=w364) -> ("error out"=w360:errorcluster, "device_type out"=w363:refnum<class "5785_2_x_1600MHz.lvclass">)  [unwired: 7 in]
            }
            n128 = Equal?(x=1, y=w329) -> (x = y?=w338:bool)
            n129 = Less Or Equal?(x=w330, y=w329) -> (x <= y?=w341:bool)
            n130 = case shown="True" w341 {
              tunnel: [w350 0 ("run number")] -> w340
              tunnel: w329 -> [w350 _]
              frame False {
              }
              frame True {
                n131 = property on="cal mode" class="Bool (strict)"("Value"=FALSE ("cal mode")) -> ()  [unwired: 2 in, 2 out]
              }
            }
            n132 = call "concatenate array.vi"("reset"=w338, "Array"=w339) -> ("appended array"=w332:cluster{"Array":dbl[], "Array":dbl[]}[])  [unwired: 9 in]
            n133 = call "concatenate array.vi"("reset"=w338, "Array"=w337) -> ("appended array"=w334:cluster{"Array":dbl[], "Array":dbl[]}[])  [unwired: 9 in]
            n134 = Build Array (concatenate)(w334, w335) -> (→"delta phase(deg)":cluster{"freqency":dbl[], "Array":dbl[]}[])
            n135 = Build Array (concatenate)(w332, w333) -> (→"delta amp (dB)":cluster{"freqency":dbl[], "Array":dbl[]}[])
          }
          frame True {
            n136 = Less Or Equal?(x=w367, y=w372) -> (x <= y?=w370:bool)
            n137 = Equal?(x=1, y=w372) -> (x = y?=w374:bool)
            n138 = call "concatenate array.vi"("reset"=w374, "Array"=w375) -> ("appended array"=→"phase cal test (deg)":cluster{"Array":dbl[], "Array":dbl[]}[])  [unwired: 9 in]
            n139 = call "concatenate array.vi"("reset"=w374, "Array"=w377) -> ("appended array"=→"amp cal test(dB) 2":cluster{"Array":dbl[], "Array":dbl[]}[])  [unwired: 9 in]
            n140 = Select(t=states_for_scope."wait", s=w370, f=states_for_scope."INI scope") -> (s? t:f=w371:T1)
            "working" <- FALSE ("done")
          }
        }
      }
    }
    "state" <- w16
    "run number" <- w12
  }
  n141 = call <vilib>:"Clear Errors.vi"("error in (no error)"=w2) -> ("error out"=w1:errorcluster)  [unwired: 5 in, 1 out]
  n142 = call <vilib>:"Simple Error Handler.vi"("error in (no error)"=w1) -> ()  [unwired: 4 in, 5 out]
